vi "graphs+waveforms.vi"() -> ()   [LabVIEW 2023]
panel:
  out "Waveform Graph":dbl[](graph)
  in  "stop":bool
  out "Waveform Chart":dbl(graph)
  in  "Slide":dbl(slide) scale=0.0..200.0
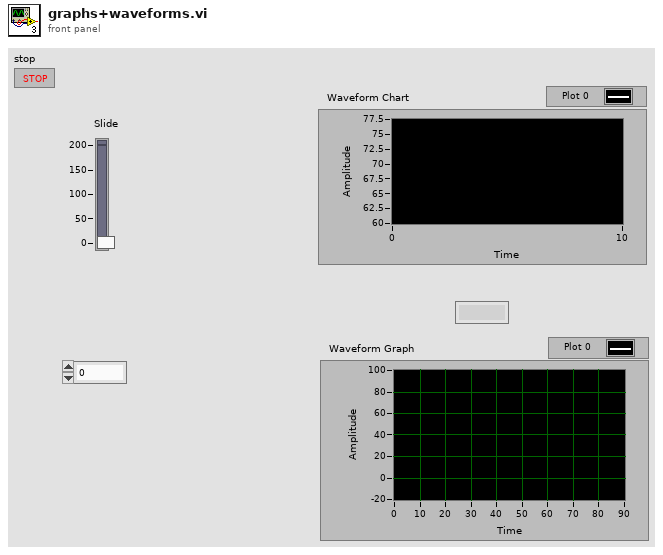
[diagram p1: front panel]
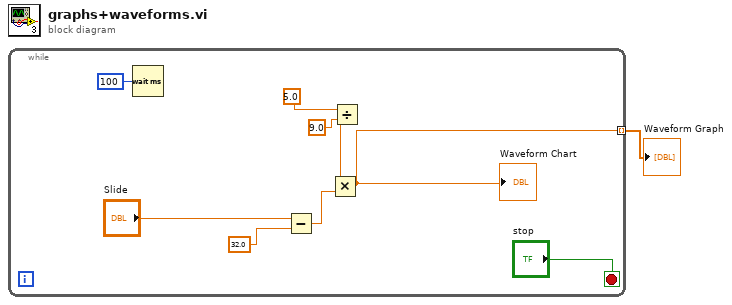
[diagram p0: block diagram]
diagram:
  n1 = while {
    tunnel: [w2] -> w1 mode=indexing
    stop <- "stop" stop-if-true
    n2 = Wait (ms)(milliseconds to wait=u32 100) -> ()  [unwired: 1 out]
    n3 = Subtract(x="Slide", y=32.0) -> (x-y=w7:dbl)
    n4 = Divide(x=5.0, y=9.0) -> (x/y=w8:dbl)
    n5 = Multiply(x=w8, y=w7) -> (x*y=w2:dbl)
    "Waveform Chart" <- w2
  }
  "Waveform Graph" <- w1
